vi "Engine-RPC-Init.vi"(8 "Error In":errorcluster, 11 "DSI Reference":refnum<class "DCM-DSI.lvclass">) -> (0 "Error Out":errorcluster, 1 "Control Mode":T1, 3 "DSI Reference":refnum<class "DCM-DSI.lvclass">)   [LabVIEW 2016, in "DSI-RT.lvlib"]
uses:
  DSI-RT.lvlib
  Shared/Typedefs/Engine-RPC-Modes.ctl
  Classes/DCM-DSI/DCM-DSI.lvclass
  <vilib>/addons/Software Calibration Management/xSCM/CalPoint.xnode
  <vilib>/addons/Software Calibration Management/xSCM/FaultPoint.xnode
  <vilib>/addons/Software Calibration Management/xSCM/ni_scm.dll
  Shared/DSI-Shared.lvlib
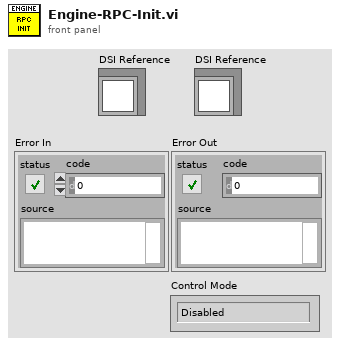
[diagram p1: front panel]
types:
  T1 = typedef "DSI-Shared.lvlib/Engine-RPC-Modes.ctl" = enum8{"Disabled", "DSI - PWM Pumps", "DSI - Sync Pumps", "User Plugin"}
  T2 = enum8{"Disabled", "DSI - PWM Pumps", "DSI - Sync Pumps", "User Plugin"}
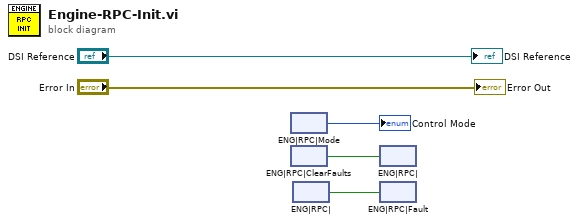
[diagram p0: block diagram]
diagram:
  n1 = xnode "ENG|RPC|Mode"() -> ("Value"=→"Control Mode":T2)
  n2 = xnode "ENG|RPC|ClearFaults"() -> ("Value"=w3:bool)
  n3 = xnode "ENG|RPC|"() -> ("Fault"=w2:bool)
  n4 = xnode "ENG|RPC|"("Clear (T)"=w3) -> ()
  n5 = xnode "ENG|RPC|Fault"("Value"=w2) -> ()
  "Error Out" <- "Error In"
  "DSI Reference" <- "DSI Reference"
